vi "run_experiment.vi"(0 "GUI refnum cluster":T34, 1 "all settings":T1={"Variable Settings"={"Measurements per Iteration"=0, "Local Data Path"=path "", "Experiment description suffix for filename (no spaces please)"="", "Network Data Path"=path "", "Copy data to network"=FALSE, "Measurement Timeout (ms)"=0, "Independent Variables"=[], "Dependent Variables"=[], "Run Test Mode"=FALSE}, "HSDIO Settings"={"Enable HSDIO Pulses"=TRUE, "Resource Name"="PXI1Slot6", "Clock Rate"=20000000.0, "Array of Script Triggers"=[], "Channels Control"=[["Hex 3D MOT b0", "1", "0", "", "", "", "", "", "", "", "", "", "", "", "", "", "", "", "", ""], ["Hex 3D MOT b0", "1", "0", "", "", "", "", "", "", "", "", "", "", "", "", "", "", "", "", ""], ["repumper bit0", "1", "0", "", "", "", "", "", "", "", "", "", "", "", "", "", "", "", "", ""], ["Trap Array beam switch", "1", "0", "", "", "", "", "", "", "", "", "", "", "", "", "", "", "", "", ""], ["2D MOT switch", "1", "0", "", "", "", "", "", "", "", "", "", "", "", "", "", "", "", "", ""], ["Hamamatsu CCD trigger", "1", "0", "", "", "", "", "", "", "", "", "", "", "", "", "", "", "", "", ""], ["Luca CCD trigger", "1", "0", "", "", "", "", "", "", "", "", "", "", "", "", "", "", "", "", ""], ["broken", "", "", "", "", "", "", "", "", "", "", "", "", "", "", "", "", "", "", ""], ["repumper bit1", "1", "0", "", "", "", "", "", "", "", "", "", "", "", "", "", "", "", "", ""], ["blow away", "1", "0", "", "", "", "", "", "", "", "", "", "", "", "", "", "", "", "", ""], ["trap shutter", "1", "0", "", "", "", "", "", "", "", "", "", "", "", "", "", "", "", "", ""], ["1038 switch", "1", "0", "", "", "", "", "", "", "", "", "", "", "", "", "", "", "", "", ""], ["", "", "", "", "", "", "", "", "", "", "", "", "", "", "", "", "", "", "", ""], ["", "", "", "", "", "", "", "", "", "", "", "", "", "", "", "", "", "", "", ""], ["", "", "", "", "", "", "", "", "", "", "", "", "", "", "", "", "", "", "", ""], ["", "", "", "", "", "", "", "", "", "", "", "", "", "", "", "", "", "", "", ""], ["", "", "", "", "", "", "", "", "", "", "", "", "", "", "", "", "", "", "", ""], ["", "", "", "", "", "", "", "", "", "", "", "", "", "", "", "", "", "", "", ""], ["", "", "", "", "", "", "", "", "", "", "", "", "", "", "", "", "", "", "", ""], ["", "", "", "", "", "", "", "", "", "", "", "", "", "", "", "", "", "", "", ""], ["", "", "", "", "", "", "", "", "", "", "", "", "", "", "", "", "", "", "", ""], ["", "", "", "", "", "", "", "", "", "", "", "", "", "", "", "", "", "", "", ""], ["", "", "", "", "", "", "", "", "", "", "", "", "", "", "", "", "", "", "", ""], ["", "", "", "", "", "", "", "", "", "", "", "", "", "", "", "", "", "", "", ""], ["", "", "", "", "", "", "", "", "", "", "", "", "", "", "", "", "", "", "", ""], ["", "", "", "", "", "", "", "", "", "", "", "", "", "", "", "", "", "", "", ""], ["", "", "", "", "", "", "", "", "", "", "", "", "", "", "", "", "", "", "", ""], ["", "", "", "", "", "", "", "", "", "", "", "", "", "", "", "", "", "", "", ""], ["", "", "", "", "", "", "", "", "", "", "", "", "", "", "", "", "", "", "", ""], ["", "", "", "", "", "", "", "", "", "", "", "", "", "", "", "", "", "", "", ""], ["", "", "", "", "", "", "", "", "", "", "", "", "", "", "", "", "", "", "", ""]], "Pulse Generation Script"="script script1\n     Generate RedTrap_compress_temp\nend script", "Start Trigger"={"Wait for start trigger?"=FALSE, "source (PFI 0)"="PFI0", "edge (rising)"=12}, "Hardware alignment quantum\n(in samples)"=1, "Inital State"="", "Idle State"="", "Active Channels"="", "Array of Waveforms"=[]}, "DAQmx Pulse Settings"={"Enable DAQmx Pulses"=FALSE, "DAQmx Physical Channels"="", "Clock Rate"=0.0, "units/sec (ms=1000)"=0.0, "Start Trigger"={"Wait for start trigger?"=FALSE, "source"="", "edge"=0}, "Timing Sequence Control"=[]}, "DDS Settings"={"Enable DDS"=FALSE, "Array of DDS Boxes"=[]}, "Camera settings"={"Analog Gain (0-5)"=4, "Exposure Time"=0.01, "EM Gain (0-255)"=0, "Trigger Polarity"="ATP P", "External Trigger Mode"="EMD E", "Scan Speed"="SSP H", "External Trigger Source"="ESC B", "Scan Mode"="SMD N", "Super Pixel Binning\n(if enabled in Scan Mode)"="SPX 1", "Camera Sub-array acquisition region\n(if enabled in scan mode)"={"Left"=0, "Top"=0, "Width"=0, "Height"=0}, "Use camera?"=FALSE, "# image buffers"=100, "shots per measurement"=100, "Force images to U16"=FALSE, "Low Light Sensitivity"="LLS 0", "cooling"="CSW F", "fan"="FAN F", "Frame Grabber acquisition region"={"Left"=0, "Top"=0, "Right"=0, "Bottom"=0}}, "Counter Settings"={"Enable Counters"=FALSE, "Array of Counter Settings"=[]}, "Filter Cluster"={"Counter Filter thresholds"=[], "Data Filters\nROI Minimum Thresholds"=[]}, "Analog Output Parameters"={"Enable Analog Out?"=FALSE, "Physical Channel"="PXI1Slot2/ao0:2", "Minimum Value"=-10.0, "Maximum Value"=10.0, "Samples per second"=0.0, "Total AO Time (seconds)"=0.0, "Start Trigger"={"Wait for start trigger?"=FALSE, "source"="/Dev1/PFI0", "edge"=10280}, "Analog Output Waveforms (channel, time)"=[]}, "Notes"="", "HP83623A Generator Settings Array"=[], "Iteration Graph Settings"={"Plot Regions"="", "Plot Shots"=""}, "PI Piezo Settings"={"Enable"=FALSE, "Array of Piezo Controllers"=[]}, "Andor settings"={"Andor Path"=path "", "Copy any Andor files"=FALSE, "Wait time before copying Andor files (ms)"=0}, "Measurement Chart Settings"={"Which regions to plot (comma separated)"="", "Which shot to plot"=0}, "HP8662A Synthesized Signal Generator Array"=[], "HP83712B Synthesized CW Generator Array"=[], "TTL input"={"Enable"=FALSE, "lines"=""}} {"Variable Settings"."Independent Variables"."# steps" min=1 step=1; "Variable Settings"."Measurements per Iteration" min=1 step=1; "HSDIO Settings"."Hardware alignment quantum\n(in samples)" min=1 step=1; "HSDIO Settings"."Array of Script Triggers"."level" items=["High Level"=34, "Low Level"=35]; "HSDIO Settings"."Array of Script Triggers"."edge" items=["Rising Edge"=12, "Falling Edge"=13]; "HSDIO Settings"."Start Trigger"."edge (rising)" items=["Rising Edge"=12, "Falling Edge"=13]; "HSDIO Settings"."Clock Rate" min=0.0 max=200000000.0 format="%.2p"; "DAQmx Pulse Settings"."Start Trigger"."edge" items=["Rising"=10280, "Falling"=10171]; "DAQmx Pulse Settings"."Clock Rate" min=0.0 max=200000000.0 format="%.2p"; "Camera settings"."Frame Grabber acquisition region"."Bottom" max=512 step=1; "Camera settings"."Frame Grabber acquisition region"."Right" max=512 step=1; "Camera settings"."Frame Grabber acquisition region"."Top" max=512 step=1; "Camera settings"."Frame Grabber acquisition region"."Left" max=512 step=1; "Camera settings"."shots per measurement" min=0 step=1; "Camera settings"."# image buffers" min=0 step=1; "Camera settings"."Camera Sub-array acquisition region\n(if enabled in scan mode)"."Height" min=16 max=512 step=16; "Camera settings"."Camera Sub-array acquisition region\n(if enabled in scan mode)"."Width" min=16 max=512 step=16; "Camera settings"."Camera Sub-array acquisition region\n(if enabled in scan mode)"."Top" max=496 step=16; "Camera settings"."Camera Sub-array acquisition region\n(if enabled in scan mode)"."Left" max=496 step=16; "Camera settings"."Analog Gain (0-5)" max=5 step=1; "Counter Settings"."Array of Counter Settings"."Binwidth (ms)" format="%0.2f"; "Analog Output Parameters"."Start Trigger"."edge" items=["Rising"=10280, "Falling"=10171]; "Analog Output Parameters"."Maximum Value" format="%0.2f"; "Analog Output Parameters"."Minimum Value" format="%0.2f"}, 2 "Variable Settings Refnum":refnum<vi>, 7 "error in (no error)":errorcluster, 8 "Image Display Refnum Array":refnum<vi>[](array[refnum]), 12 "Camera Temperature Refnum":refnum<vi>, 14 "HSDIO Status Refnum":refnum<vi>, 16 "# intervals (mutli-shot)":i32=128, 17 "Notes Refnum":refnum<vi>, 22 "Hamamatsu_C9100-13.lvclass":refnum<class "Hamamatsu_C9100-13.lvclass">) -> (20 "Array of ROI sums":dbl[][][][](array[numeric])=[[[[-878.86977886979]]]], 21 "Image Array for whole experiment":T39[][][](array[plugin-control]) caption="(Cycles, Iterations, Measurements, Shots, scaling above)", 23 "Histogram of ROI Sum over All Images for last ROI":T37, 24 "Average of All Images from experiment":T39(plugin-control) caption="Average of All Images (dynamically scaled)", 25 "Camera out":refnum<class "Hamamatsu_C9100-13.lvclass">, 27 "error out":errorcluster)   [LabVIEW 2013]
doc: "I Description:\nThis example uses a script to manage the generation of a dynamic pattern at a specified clock rate.\n\nII Instructions for Running:\n1. Enter the digital channels on the hardware device to generate digital pattern in the Channel List control.\n2. Specify the clock rate for the generation in the Clock Rate control.\n3. Click the Stop button when you want to stop the generation\n\nIII Block Diagram Steps:\n1. Initialize for a generation session.\n2. Assign specified channels in Channel List for dynamic operation.\n3. Configure the Sample clock to use the onboard clock, and configure the clock rate.\n4. Set the generation mode to Scripted.\n5. Query the Data Width property to determine which Write function to use.\nNote: Different devices have different default values for the Data Width property. If you know the Data Width of your device, you may omit the property node and case structure.\n6. Write digital patterns to the onboard memory of the digital device.\n7. Write the script to the onboard memory.\n8. Initiate dynamic pattern generation.\n9. Wait until the Stop button is clicked or an error occurs, and exit the While loop. \n The niHSDIO Is Done VI is used in the while loop to check only for errors.\n10. Abort generation and close the session.\n\nIV I/O Connections Overview:\nMake connections from output terminals to match the channels specified by Channel List. In this example, the digital pattern is generated from the first 16 digital channels of the device."
uses:
  Camera/Hamamatsu_C9100-13/Hamamatsu_C9100-13.lvclass
  ExperimentVariables/ExperimentVariables.lvclass
  DDS/DDS.lvclass
  PI_piezo/PI_Piezo.lvclass
  HSDIO/HSDIO.lvclass
  DAQmx_pulse_out/DAQmx_pulse_out.lvclass
  Analog_output/Analog_Output.lvclass
  Counter/Counter.lvclass
  GPIB/GPIB.lvclass
  TTL_input/TTL_input.lvclass
  Analog_output/AO_settings.ctl
  Camera/Hamamatsu_C9100-13/camera_setup.ctl
  DDS drivers v3/DDS RAM mode.ctl
  <vilib>/ni845x/ni845x.llb/ni845xControl.ctl
  <instrlib>/niHSDIO/niHSDIO.llb/niHSDIO_ctl Trigger Script - trigID Values (Ring).ctl
  <instrlib>/niHSDIO/niHSDIO.llb/niHSDIO_ctl Trigger DigEdge - Edge Values (Ring).ctl
  <instrlib>/niHSDIO/niHSDIO.llb/niHSDIO_ctl Trigger Source Values (Ring).ctl
  ExperimentVariables/Variable_Settings.ctl
  Counter/Counter_Settings_Control.ctl
  HSDIO/HSDIO_settings.ctl
  DAQmx_pulse_out/settings.ctl
  <instrlib>/niHSDIO/niHSDIO.llb/niHSDIO_ctl Trigger DigLvl - Level Values (Ring).ctl
  histogram.ctl
  gui_refnum.ctl
  Counter/counter_graph_refnums.ctl
  filters/filters.ctl
  gui_execution_controls.ctl
  DDS drivers v3/Array_of_DDS_Boxes.ctl
  DDS drivers v3/DDS_box_device_reference.ctl
  DDS drivers v3/DDS_box_cluster.ctl
  DDS/DDS_Settings_Cluster.ctl
  config_file_io/all_settings.ctl
  GPIB/HP83623A_RF_Generator/HP83623A_array.ctl
  GPIB/HP83623A_RF_Generator/HP83623A_RF_Generator.lvclass
  PI_piezo/settings.ctl
  PI_piezo/status.ctl
  Camera/Andor/Andor_settings.ctl
  gui/measurement_graph.ctl
  GPIB/RF_Generator_settings.ctl
  GPIB/RF_Generator_settings_array.ctl
  DDS drivers v3/DDS_profile.ctl
  DDS drivers v3/DDS_channel.ctl
  DDS drivers v3/array_of_DDS_profiles.ctl
  DDS drivers v3/array_of_DDS_channels.ctl
  TTL_input/TTL_input_settings.ctl
  HSDIO/waveform.ctl
  PI_piezo/piezo_channel.ctl
  PI_piezo/piezo_controller.ctl
  GPIB/HP83623A_RF_Generator/HP83623A.ctl
panel:
  out "Counter out":refnum<class "Counter.lvclass">
  out "HSDIO":refnum<class "HSDIO.lvclass">
  out "Run Test Mode":bool
  in  "Tab Control":T38(tab)=enum."Filters"
  # "Parameters will be evaluated once at the beginning of the experiment from top to bottom, \nso any parameter may depend on all those above it.\nVariables will be evaluated each iteration.\nParameters and Variables may be used in various other experiment settings, as noted.\nSee LabView Help -> Formula Node and Expression Node Functions for a list of available functions."
  # "Parameters will be evaluated once at the beginning of the experiment from top to bottom, \nso any parameter may depend on all those above it.\nVariables will be evaluated each iteration.\nParameters and Variables may be used in various other experiment settings, as noted.\nSee LabView Help -> Formula Node and Expression Node Functions for a list of available functions."
  # "Regions of Interest -->"
  # "Shots\n   |\n  V"
  # "Counters -->"
  # "Counter\n    bins\n       |\n      V"
  # "Notes will be auto-evaluated and will be saved with comments in each experiment directory."
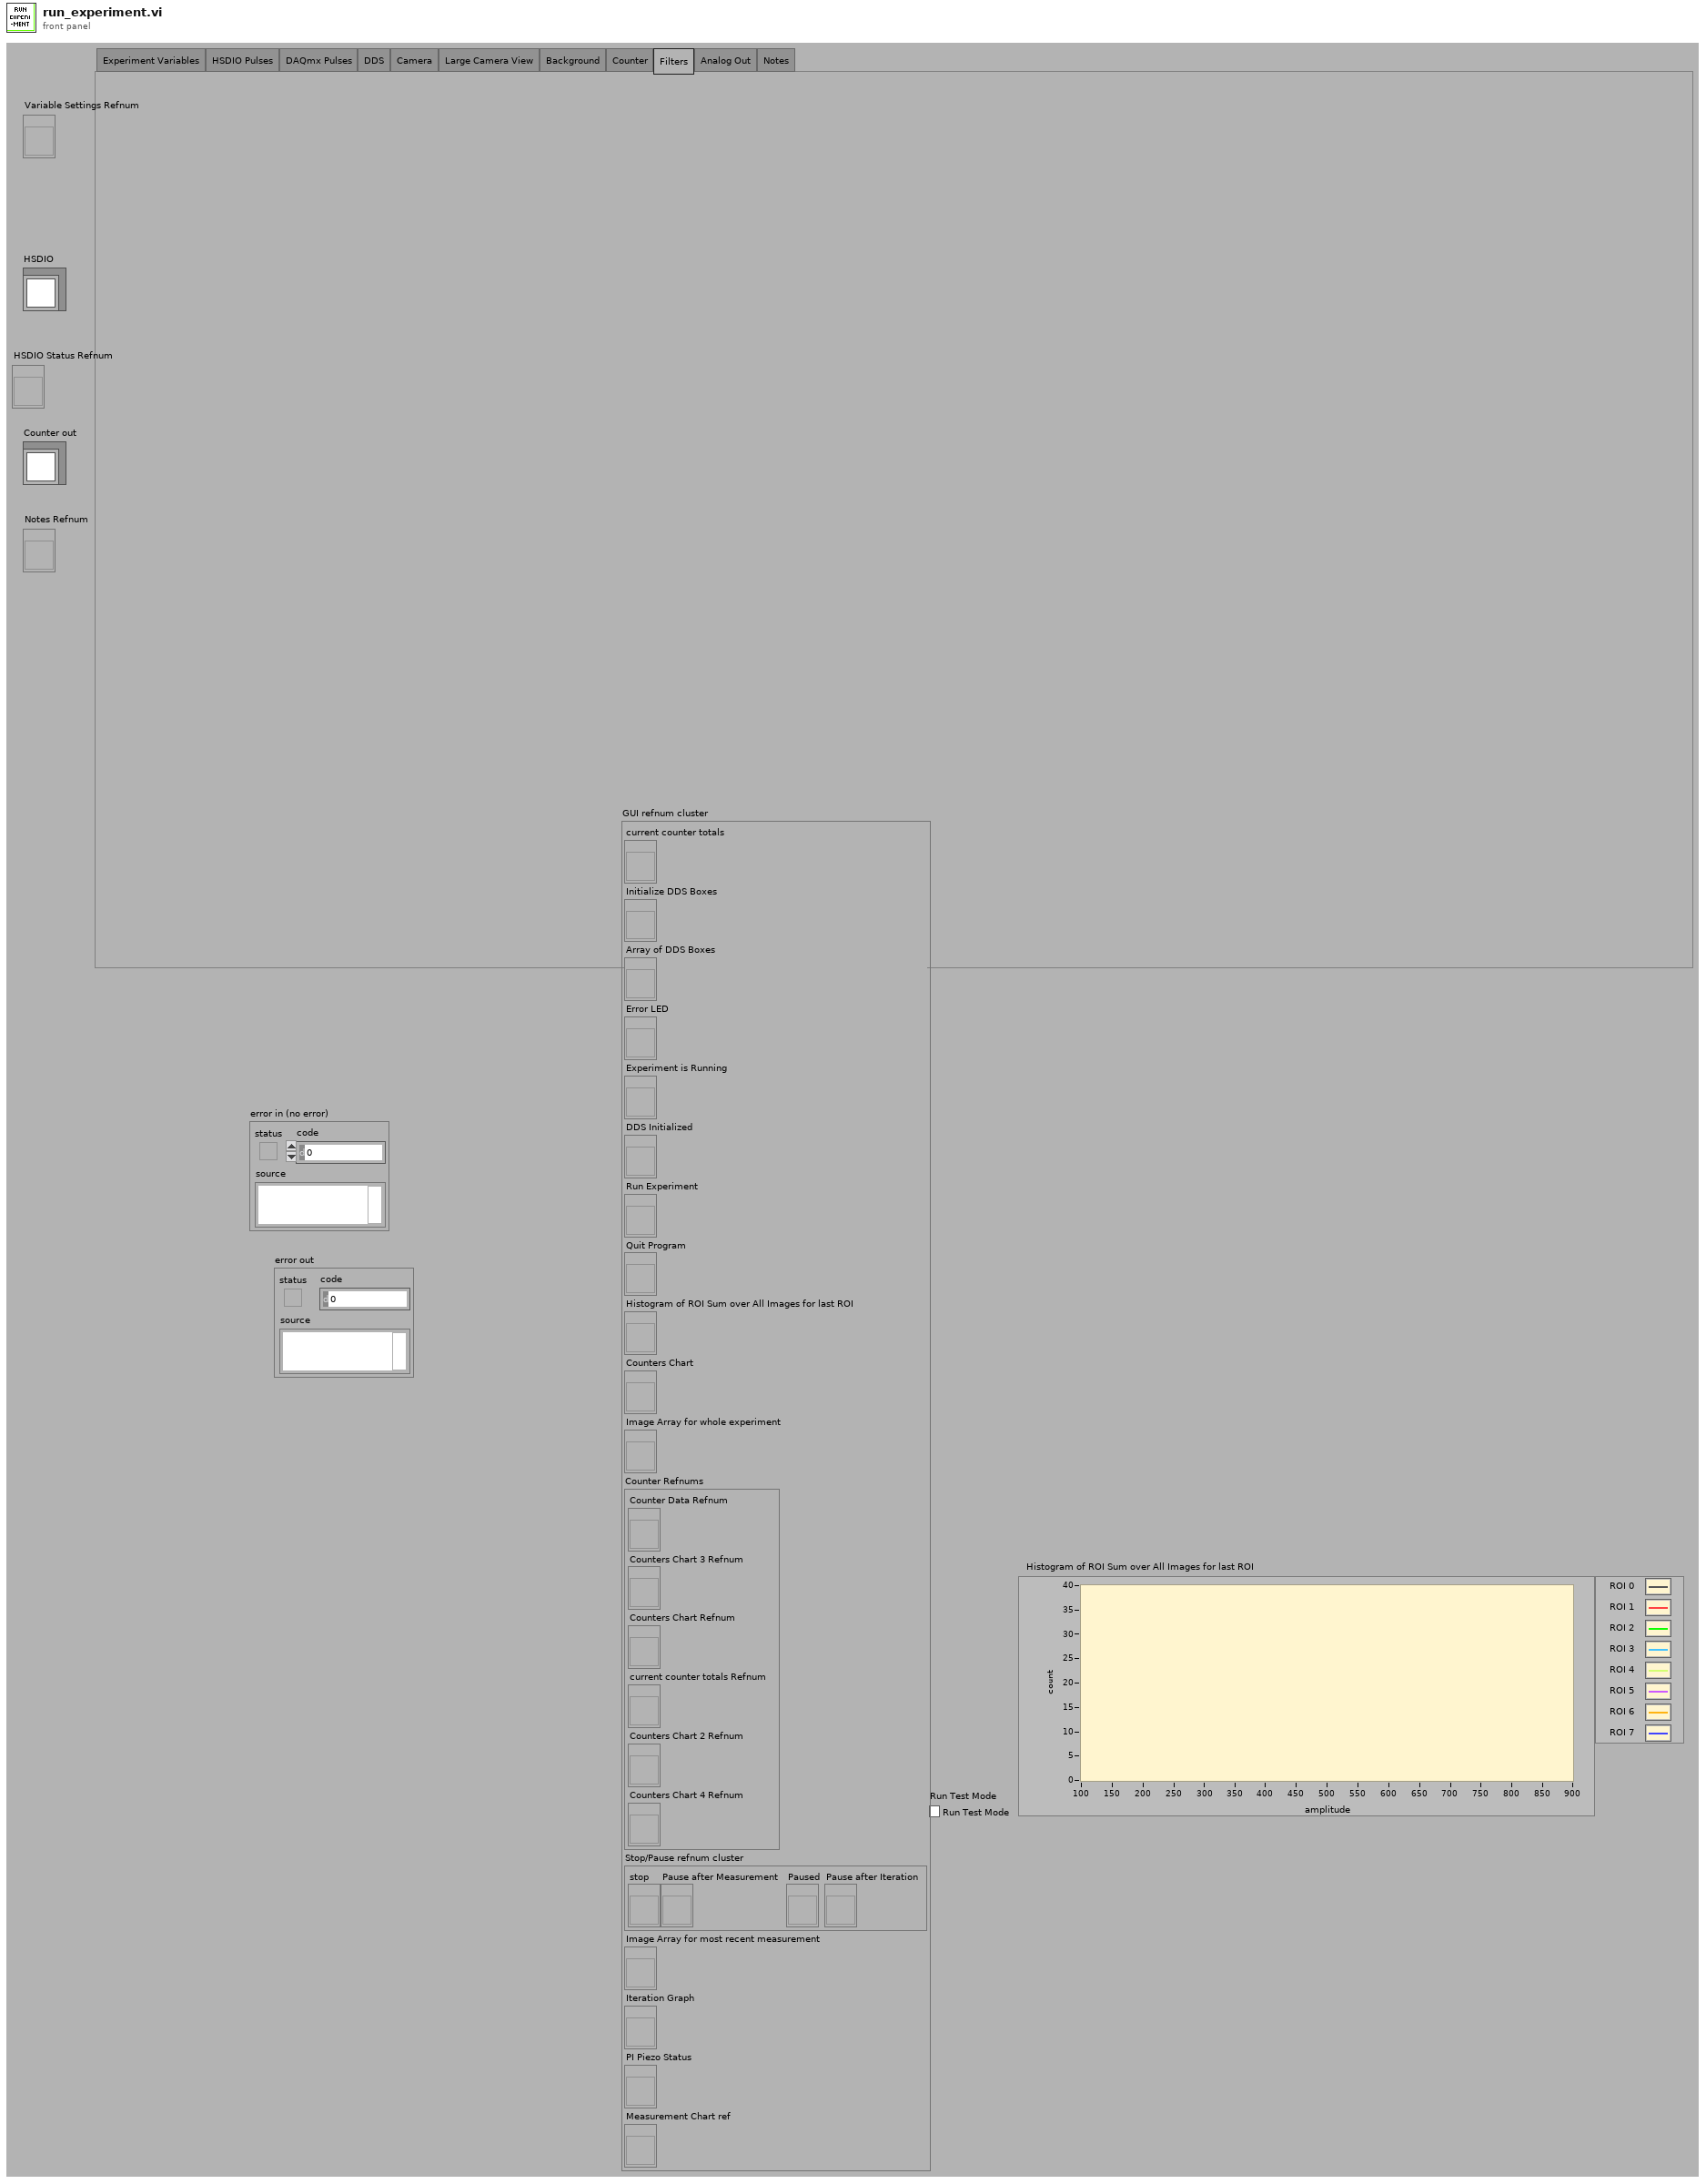
[diagram p1: front panel]
types:
  T1 = typedef "all_settings.ctl" = cluster{"Variable Settings":T2, "HSDIO Settings":T3, "DAQmx Pulse Settings":T9, "DDS Settings":T10, "Camera settings":T20, "Counter Settings":T21, "Filter Cluster":T22, "Analog Output Parameters":T23, "Notes":string, "HP83623A Generator Settings Array":T24, "Iteration Graph Settings":cluster{"Plot Regions":string, "Plot Shots":string}, "PI Piezo Settings":T26, "Andor settings":T29, "Measurement Chart Settings":T30, "HP8662A Synthesized Signal Generator Array":T31, "HP83712B Synthesized CW Generator Array":T31, "TTL input":T33}
  T2 = typedef "ExperimentVariables.lvclass/Variable_Settings.ctl" = cluster{"Measurements per Iteration":i32, "Local Data Path":path, "Experiment description suffix for filename (no spaces please)":string, "Network Data Path":path, "Copy data to network":bool, "Measurement Timeout (ms)":u32, "Independent Variables":cluster{"Description":string, "Name (a,a0...a9)":string, "min":dbl, "max":dbl, "# steps":u32}[], "Dependent Variables":cluster{"Description":string, "Name (a,a0...a9)":string, "Equation":string, "Result":dbl}[], "Run Test Mode":bool}
  T3 = typedef "HSDIO.lvclass/HSDIO_settings.ctl" = cluster{"Enable HSDIO Pulses":bool, "Resource Name":refnum<k15>, "Clock Rate":dbl, "Array of Script Triggers":cluster{"trigger id (script trigger 0)":T4, "source (PFI 0)":T5, "Trigger Type":enum32{"Edge", "Level"}, "edge":T6, "level":T7}[], "Channels Control":string[][], "Pulse Generation Script":string, "Start Trigger":cluster{"Wait for start trigger?":bool, "source (PFI 0)":T5, "edge (rising)":T6}, "Hardware alignment quantum\n(in samples)":u16, "Inital State":string, "Idle State":string, "Active Channels":string, "Array of Waveforms":T8[]}
  T4 = typedef "niHSDIO_ctl Trigger Script - trigID Values (Ring).ctl" = string
  T5 = typedef "niHSDIO_ctl Trigger Source Values (Ring).ctl" = string
  T6 = typedef "niHSDIO_ctl Trigger DigEdge - Edge Values (Ring).ctl" = i32
  T7 = typedef "niHSDIO_ctl Trigger DigLvl - Level Values (Ring).ctl" = i32
  T8 = typedef "HSDIO.lvclass/waveform.ctl" = cluster{"name":string, "transitions":u32[], "states":u8[][]}
  T9 = typedef "DAQmx_pulse_out.lvclass/settings.ctl" = cluster{"Enable DAQmx Pulses":bool, "DAQmx Physical Channels":tag, "Clock Rate":dbl, "units/sec (ms=1000)":dbl, "Start Trigger":cluster{"Wait for start trigger?":bool, "source":tag, "edge":i32}, "Timing Sequence Control":string[][]}
  T10 = typedef "DDS_Settings_Cluster.ctl" = cluster{"Enable DDS":bool, "Array of DDS Boxes":T11}
  T11 = typedef "Array_of_DDS_Boxes.ctl" = T12[]
  T12 = typedef "DDS_box_cluster.ctl" = cluster{"DDS box device reference":T13, "Array of DDS Channels (4)":T15, "Enable":bool, "Description":string}
  T13 = typedef "DDS_box_device_reference.ctl" = cluster{"NI USB-8451 device reference":T14, "DIO port":u8, "Serial Clock Rate [kHz]":u16}
  T14 = typedef "ni845xControl.ctl" = refnum<k21>
  T15 = typedef "DDS.lvclass/array_of_DDS_channels.ctl" = T16[]
  T16 = typedef "DDS.lvclass/DDS_channel.ctl" = cluster{"Power":bool, "Channel Parameters":cluster{"Ref Clock Rate [kHz]":dbl, "Full Scale Output\nPower [dBm]":dbl}, "RAM Enable":bool, "RAM Dest Type":u8, "RAM Default":cluster{"Frequency [MHz]":dbl, "Amplitude [dBm]":dbl, "Phase Offset [rad]":dbl}, "Array of DDS Profiles (8)":T17, "Description":string}
  T17 = typedef "DDS.lvclass/array_of_DDS_profiles.ctl" = T18[]
  T18 = typedef "DDS_profile.ctl" = cluster{"Single Tone":cluster{"Frequency [MHz]":dbl, "Amplitude [dBm]":dbl, "Phase Offset [rad]":dbl}, "RAM Mode ":T19, "Zero-crossing":bool, "No Dwell High":bool, "Function/Static":bool, "RAM Function Settings":string[], "RAM Static Array":dbl[], "Description":string}
  T19 = typedef "DDS RAM mode.ctl" = enum16{"Direct Switch", "Ramp Up", "Bidirectional Ramp", "Continuous Bidirectional Ramp", "Continuous Recirculate", "Direct Switch 2", "Direct Switch 3", "Direct Switch 4"}
  T20 = typedef "Hamamatsu_C9100-13.lvclass/camera_setup.ctl" = cluster{"Analog Gain (0-5)":u8, "Exposure Time":dbl, "EM Gain (0-255)":u8, "Trigger Polarity":string, "External Trigger Mode":string, "Scan Speed":string, "External Trigger Source":string, "Scan Mode":string, "Super Pixel Binning\n(if enabled in Scan Mode)":string, "Camera Sub-array acquisition region\n(if enabled in scan mode)":cluster{"Left":u16, "Top":u16, "Width":u16, "Height":u16}, "Use camera?":bool, "# image buffers":i32, "shots per measurement":i32, "Force images to U16":bool, "Low Light Sensitivity":string, "cooling":string, "fan":string, "Frame Grabber acquisition region":cluster{"Left":i32, "Top":i32, "Right":i32, "Bottom":i32}}
  T21 = typedef "Counter.lvclass/Counter_Settings_Control.ctl" = cluster{"Enable Counters":bool, "Array of Counter Settings":cluster{"Counter Channel":tag, "Time-Bin Clock Channel":tag, "Binwidth (ms)":dbl}[]}
  T22 = typedef "filters.ctl" = cluster{"Counter Filter thresholds":u32[][], "Data Filters\nROI Minimum Thresholds":u64[][]}
  T23 = typedef "Analog_Output.lvclass/AO_settings.ctl" = cluster{"Enable Analog Out?":bool, "Physical Channel":tag, "Minimum Value":dbl, "Maximum Value":dbl, "Samples per second":dbl, "Total AO Time (seconds)":dbl, "Start Trigger":cluster{"Wait for start trigger?":bool, "source":tag, "edge":i32}, "Analog Output Waveforms (channel, time)":dbl[][]}
  T24 = typedef "HP83623A_RF_Generator.lvclass/HP83623A_array.ctl" = T25[]
  T25 = typedef "HP83623A_RF_Generator.lvclass/HP83623A.ctl" = cluster{"Frequency (Hz)":dbl, "Power (dBm)":dbl, "Enabled":bool, "initialized":bool, "RF Output On/Off":bool, "External Trigger?":bool, "VISA Session":refnum<visa-resource-name>, "Generator Name":string}
  T26 = typedef "PI_Piezo.lvclass/settings.ctl" = cluster{"Enable":bool, "Array of Piezo Controllers":T27[]}
  T27 = typedef "PI_Piezo.lvclass/piezo_controller.ctl" = cluster{"Enable":bool, "Serial No.":string, "Array of Piezo Channels":T28[]}
  T28 = typedef "PI_Piezo.lvclass/piezo_channel.ctl" = cluster{"Servo":bool, "Set Position":dbl}
  T29 = typedef "Andor_settings.ctl" = cluster{"Andor Path":path, "Copy any Andor files":bool, "Wait time before copying Andor files (ms)":u16}
  T30 = typedef "measurement_graph.ctl" = cluster{"Which regions to plot (comma separated)":string, "Which shot to plot":u8}
  T31 = typedef "GPIB.lvclass/RF_Generator_settings_array.ctl" = T32[]
  T32 = typedef "GPIB.lvclass/RF_Generator_settings.ctl" = cluster{"Enable":bool, "Description":string, "GPIB channel #":u8, "Frequency (MHz)":dbl, "Power (dBm)":dbl}
  T33 = typedef "TTL_input.lvclass/TTL_input_settings.ctl" = cluster{"Enable":bool, "lines":tag}
  T34 = typedef "gui_refnum.ctl" = cluster{"current counter totals":refnum<vi>, "Initialize DDS Boxes":refnum<vi>, "Array of DDS Boxes":refnum<vi>, "Error LED":refnum<vi>, "Experiment is Running":refnum<vi>, "DDS Initialized":refnum<vi>, "Run Experiment":refnum<vi>, "Quit Program":refnum<vi>, "Histogram of ROI Sum over All Images for last ROI":refnum<vi>, "Counters Chart":refnum<vi>, "Image Array for whole experiment":refnum<vi>, "Counter Refnums":T35, "Stop/Pause refnum cluster":T36, "Image Array for most recent measurement":refnum<vi>, "Iteration Graph":refnum<vi>, "PI Piezo Status":refnum<vi>, "Measurement Chart ref":refnum<vi>}
  T35 = typedef "counter_graph_refnums.ctl" = cluster{"Counter Data Refnum":refnum<vi>, "Counters Chart 3 Refnum":refnum<vi>, "Counters Chart Refnum":refnum<vi>, "current counter totals Refnum":refnum<vi>, "Counters Chart 2 Refnum":refnum<vi>, "Counters Chart 4 Refnum":refnum<vi>}
  T36 = typedef "gui_execution_controls.ctl" = cluster{"stop":refnum<vi>, "Pause after Measurement":refnum<vi>, "Paused":refnum<vi>, "Pause after Iteration":refnum<vi>}
  T37 = typedef "histogram.ctl" = cluster{"X Values":dbl[], "Histogram: h(x)":i32[]}[]
  T38 = enum32{"Experiment Variables", "HSDIO Pulses", "DAQmx Pulses", "DDS", "Camera", "Large Camera View", "Background", "Counter", "Filters", "Analog Out", "Notes"}
  T39 = typedef "IMAQ Image.ctl" = refnum<image>
  T40 = enum16{"reset", "experiment start", "experiment end", "quit"}
  T41 = cluster{"Plot Regions":string, "Plot Shots":string}
  T42 = cluster{"X Values":dbl[], "Histogram: h(x)":i32[]}[]
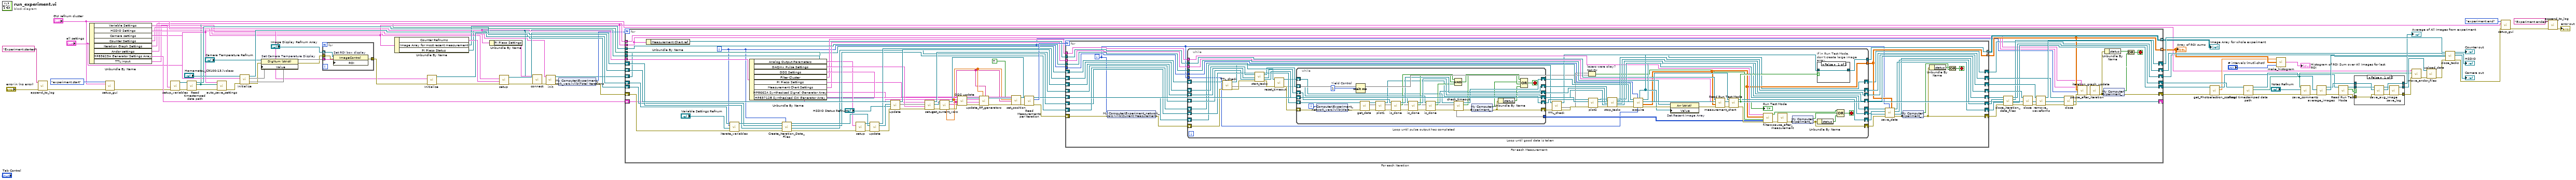
[diagram p0: block diagram]
diagram:
  n1 = call "append_to_log.vi"("error in"="error in (no error)", "string"="Experiment started") -> ("error out"=w58:errorcluster)  [unwired: 9 in]
  n2 = Unbundle By Name("all settings") -> ("Variable Settings"=w25:T2, "HSDIO Settings"=w24:T3, "Camera settings"=w23:T20, "Counter Settings"=w22:T21, "Iteration Graph Settings"=w19:T41, "Andor settings"=w11:T29, "HP83623A Generator Settings Array"=w9:T24, "TTL input"=w5:T33)
  n3 = call "setup_gui.vi"("Enum"=T40."experiment start", "GUI refnum cluster"="GUI refnum cluster", "error in (no error)"=w58) -> ("error out"=w8:errorcluster)  [unwired: 12 in]
  n4 = call "setup_variables.vi"("error in (no error)"=w8, "Variable Settings"=w25) -> ("error out"=w45:errorcluster, "ExperimentVariables out"=w47:refnum<class "ExperimentVariables.lvclass">)  [unwired: 8 in]
  n5 = call-dynamic "Read timestamped data path.vi"("error in (no error)"=w45, "ExperimentVariables in"=w47) -> ("error out"=w26:errorcluster, "Specific Data Files Path"=w14:path, "ExperimentVariables out"=w46:refnum<class "ExperimentVariables.lvclass">)  [unwired: 7 in]
  n6 = call "auto_save_settings.vi"("error in"=w26, "base path"=w14, "all settings"="all settings") -> ("error out"=w21:errorcluster)  [unwired: 8 in]
  n7 = call-dynamic "initialize.vi"("error in (no error)"=w21, 10:w23, "Hamamatsu_C9100-13 in"="Hamamatsu_C9100-13.lvclass") -> ("error out"=w62:errorcluster, 2:w63, "Hamamatsu_C9100-13 out"=w69:refnum<class "Hamamatsu_C9100-13.lvclass">, 6:w70)  [unwired: 5 in]
  n8 = property on="Set Camera Temperature Display" class="DigNum (strict)"(reference="Camera Temperature Refnum", error in=w62, "Value"=w63) -> (error out=w61:errorcluster)  [unwired: 1 out]
  n9 = for {
    tunnel: "Image Display Refnum Array" -> [w84] mode=indexing
    tunnel: w70 -> [w83]
    tunnel: w61 -> [w82]
    tunnel: [w81] -> w71
    n10 = property on="Set ROI box display" class="ImageControl"(reference=w84, error in=w82, "ROI"=w83) -> (error out=w81:errorcluster)  [unwired: 1 out]
  }
  n11 = Unbundle By Name("GUI refnum cluster") -> ("Counter Refnums"=w28:T35, "Image Array for most recent measurement"=w27:refnum<vi>, "PI Piezo Status"=w15:refnum<vi>)
  n12 = call "Initialize.vi"("error in (no error)"=w71, 10:w24) -> ("error out"=w54:errorcluster, "HSDIO out"=w75:refnum<class "HSDIO.lvclass">)  [unwired: 8 in]
  n13 = Unbundle By Name("all settings") -> ("PI Piezo Settings"=w16:T26)
  n14 = call "setup.vi"("error in (no error)"=w54, "Counter Refnums"=w28, "Counter Settings"=w22) -> ("error out"=w18:errorcluster, "Counter out"=w53:refnum<class "Counter.lvclass">)  [unwired: 7 in]
  n15 = call "connect.vi"(0:w16, 1:w15, "error in"=w18) -> ("error out"=w4:errorcluster)  [unwired: 16 in]
  n16 = call "init.vi"("error in (no error)"=w4, "TTL input"=w5) -> ("error out"=w3:errorcluster, "TTL_input out"=w2:refnum<class "TTL_input.lvclass">)  [unwired: 8 in]
  n17 = shared-variable "My Computer\\Experiment_network_vars.lvlib\\Total Iterations"(error in=w3) -> (w7:u32, error out=w6:errorcluster)
  n18 = for "For each Iteration" {
    N: w7 -> [_]
    shift-right: [w89] -> w33
    shift-left: w6 -> [w159]
    tunnel: [w111] -> w67 mode=indexing
    shift-right: [w155] -> w76
    shift-left: w75 -> [w158]
    shift-right: [w121] -> w77
    shift-left: w53 -> [w131]
    shift-right: [w124] -> w50
    shift-left: w46 -> [w160]
    tunnel: [w136] -> w74 mode=indexing
    shift-right: [w112] -> w34
    shift-left: w69 -> [w130]
    tunnel: w27 -> [w120]
    tunnel: "all settings" -> [w119]
    tunnel: "GUI refnum cluster" -> [w101]
    tunnel: w19 -> [w108]
    tunnel: w15 -> [w106]
    tunnel: w14 -> [w102]
    shift-right: [w92] -> _
    shift-left: w9 -> [w93]
    shift-right: [w87] -> w1
    shift-left: w2 -> [w88]
    i -> [w85]
    stop <- w162 stop-if-true
    n19 = Unbundle By Name(w101) -> ("Measurement Chart ref"=w100:refnum<vi>)
    n20 = call-dynamic "iterate_variables.vi"("error in (no error)"=w159, "Variable Settings Refnum"="Variable Settings Refnum", "Current Iteration"=w85, "ExperimentVariables in"=w160) -> ("error out"=w133:errorcluster, "ExperimentVariables out"=w135:refnum<class "ExperimentVariables.lvclass">)  [unwired: 6 in]
    n21 = Unbundle By Name(w119) -> ("Analog Output Parameters"=w116:T23, "DAQmx Pulse Settings"=w117:T9, "DDS Settings"=w118:T10, "Filter Cluster"=w115:T22, "PI Piezo Settings"=w107:T26, "Measurement Chart Settings"=w99:T30, "HP8662A Synthesized Signal Generator Array"=w98:T31, "HP83712B Synthesized CW Generator Array"=w86:T31)
    n22 = call-dynamic "Create_Iteration_Data_Files.vi"("Current Iteration"=w85, "error in (no error)"=w133, "Counter (in)"=w131, "Hamamatsu_C9100-13 (in)"=w130, "ExperimentVariables in"=w135) -> ("error out"=w132:errorcluster, "Counter out"=w128:refnum<class "Counter.lvclass">, "Hamamatsu_C9100-13"=w129:refnum<class "Hamamatsu_C9100-13.lvclass">, "ExperimentVariables out"=w134:refnum<class "ExperimentVariables.lvclass">)  [unwired: 3 in]
    n23 = call "setup.vi"("error in (no error)"=w132, "Analog Output Parameters"=w116) -> ("error out"=w137:errorcluster, "Analog_Output out"=w138:refnum<class "Analog_Output.lvclass">)  [unwired: 8 in]
    n24 = call-dynamic "update.vi"("error in (no error)"=w137, "ExperimentVariables (in)"=w134, "Analog_Output in"=w138) -> ("error out"=w143:errorcluster, "ExperimentVariables"=w141:refnum<class "ExperimentVariables.lvclass">, "Analog_Output out"=w142:refnum<class "Analog_Output.lvclass">)  [unwired: 6 in]
    n25 = call-dynamic "update.vi"("error in (no error)"=w143, 9:"HSDIO Status Refnum", 10:w141, "HSDIO in"=w158) -> ("error out"=w113:errorcluster, 2:w152, "HSDIO out"=w157:refnum<class "HSDIO.lvclass">)  [unwired: 5 in]
    n26 = call "setup.vi"("error in (no error)"=w113, "DAQmx Pulse Settings"=w117, "ExperimentVariables (in)"=w152) -> ("error out"=w153:errorcluster, "ExperimentVariables"=w151:refnum<class "ExperimentVariables.lvclass">, "DAQmx_pulse_out out"=w150:refnum<class "DAQmx_pulse_out.lvclass">)  [unwired: 6 in]
    n27 = call-dynamic "get_current_vars.vi"("error in (no error)"=w153, "ExperimentVariables in"=w151) -> ("error out"=w154:errorcluster, "variables and parameter names"=w94:string[], "ExperimentVariables out"=w145:refnum<class "ExperimentVariables.lvclass">, "current variable and parameter values"=w95:dbl[])  [unwired: 4 in, 2 out]
    n28 = call "DDS update.vi"("error in (no error)"=w154, 9:w94, 10:w95, "DDS.lvclass (in)"=w118) -> ("error out"=w97:errorcluster)  [unwired: 6 in, 1 out]
    n29 = call "update_RF_generators.vi"(5:w94, 7:w95, "error in"=w97, 9:w86, 10:w98, "GPIB (in)"=w93) -> ("error out"=w96:errorcluster, "GPIB"=w92:refnum<class "GPIB.lvclass">)  [unwired: 4 in]
    n30 = call "set_position.vi"(0:w107, 1:w106, 2:w95, 3:w94, "error in"=w96, 6:w102, 8:TRUE ("Save positions?")) -> ("error out"=w105:errorcluster)  [unwired: 12 in]
    n31 = call-dynamic "Read Measurements per Iteration.vi"("error in (no error)"=w105, "ExperimentVariables in"=w145) -> ("error out"=w146:errorcluster, "Measurements per Iteration"=w147:i32, "ExperimentVariables out"=w144:refnum<class "ExperimentVariables.lvclass">)  [unwired: 7 in]
    n32 = for "For each Measurement" {
      N: w147 -> [_]
      shift-right: [w194] -> w156
      shift-left: w157 -> [w195]
      shift-right: [w170] -> w127
      shift-left: w146 -> [w168]
      tunnel: [w184] -> w136 mode=indexing
      tunnel: [w185] -> w111 mode=indexing
      shift-right: [w186] -> w140
      shift-left: w142 -> [w187]
      shift-right: [w180] -> w122
      shift-left: w128 -> [w190]
      shift-right: [w188] -> w149
      shift-left: w150 -> [w189]
      shift-right: [w177] -> w125
      shift-left: w144 -> [w169]
      shift-right: [w178] -> w123
      shift-left: w129 -> [w193]
      tunnel: w120 -> [w176]
      tunnel: w115 -> [w175]
      tunnel: w100 -> [w174]
      tunnel: w99 -> [w173]
      shift-right: [w165] -> w87
      shift-left: w88 -> [w166]
      tunnel: w85 -> [w164]
      i -> [w163]
      stop <- w191 stop-if-true
      n33 = shared-variable "My Computer\\Experiment_network_vars.lvlib\\Current Measurement"(w163, error in=w168) -> (error out=w167:errorcluster)
      n34 = while "Loop until good data is taken" {
        tunnel: [w224] -> w184
        tunnel: [w213] -> w185
        shift-right: [w251] -> w194
        shift-left: w195 -> [w253]
        shift-right: [w210] -> w182
        shift-left: w167 -> [w204]
        shift-right: [w237] -> w186
        shift-left: w187 -> [w236]
        shift-right: [w247] -> w181
        shift-left: w190 -> [w249]
        shift-right: [w243] -> w188
        shift-left: w189 -> [w246]
        shift-right: [w221] -> w183
        shift-left: w169 -> [w240]
        shift-right: [w223] -> w179
        shift-left: w193 -> [w234]
        tunnel: w176 -> [w219]
        tunnel: w175 -> [w218]
        tunnel: w174 -> [w217]
        tunnel: w173 -> [w214]
        shift-right: [w209] -> w165
        shift-left: w166 -> [w205]
        tunnel: w164 -> [w197]
        tunnel: w163 -> [w196]
        stop <- w254 stop-if-true
        n35 = call-dynamic "TTL_check.vi"("error in (no error)"=w204, "TTL_input in"=w205) -> ("error out"=w203:errorcluster, 1:w200, "TTL_input out"=w202:refnum<class "TTL_input.lvclass">)  [unwired: 7 in]
        n36 = call "start_tasks.vi"("Counter (in)"=w249, "Analog_Output in"=w236, "HSDIO (in)"=w253, "DAQmx_pulse_out (in)"=w246, "error in"=w203) -> ("Counter out"=w248:refnum<class "Counter.lvclass">, "Analog_Output"=w235:refnum<class "Analog_Output.lvclass">, "HSDIO"=w250:refnum<class "HSDIO.lvclass">, "DAQmx_pulse_out"=w245:refnum<class "DAQmx_pulse_out.lvclass">, "error out"=w242:errorcluster)  [unwired: 10 in]
        n37 = call-dynamic "reset_timeout.vi"("error in (no error)"=w242, "ExperimentVariables in"=w240) -> ("error out"=w241:errorcluster, "ExperimentVariables out"=w239:refnum<class "ExperimentVariables.lvclass">)  [unwired: 8 in]
        n38 = while "Loop until pulse output has completed" {
          shift-right: [w262] -> w208
          shift-left: w241 -> [w259]
          shift-right: [w284] -> w252
          shift-left: w250 -> [w285]
          shift-right: [w267] -> w229
          shift-left: w248 -> [w269]
          shift-right: [w282] -> w244
          shift-left: w245 -> [w283]
          shift-right: [w274] -> w238
          shift-left: w235 -> [w275]
          shift-right: [w280] -> w232
          shift-left: w239 -> [w260]
          tunnel: [w257] -> w206
          i -> [w261]
          stop <- w286 stop-if-true
          w287 = u32 1  # Yield Control
          n39 = shared-variable "My Computer\\Experiment_network_vars.lvlib\\Wait Loops"(w261, error in=w259) -> (error out=w258:errorcluster)
          n40 = Wait (ms)(milliseconds to wait=w287) -> ()  [unwired: 1 out]
          n41 = call-dynamic "get_data.vi"("error in (no error)"=w258, "Counter in"=w269) -> ("error out"=w266:errorcluster, 2:w257, "Counter out"=w268:refnum<class "Counter.lvclass">)  [unwired: 7 in]
          n42 = call-dynamic "plot1.vi"("error in (no error)"=w266, "Counter in"=w268) -> ("error out"=w265:errorcluster, "Counter out"=w267:refnum<class "Counter.lvclass">)  [unwired: 8 in]
          n43 = call-dynamic "is_done.vi"("error in (no error)"=w265, "HSDIO in"=w285) -> ("error out"=w281:errorcluster, "HSDIO is done?"=w273:bool, "HSDIO out"=w284:refnum<class "HSDIO.lvclass">)  [unwired: 7 in]
          n44 = call-dynamic "is_done.vi"("error in (no error)"=w281, "DAQmx_pulse_out in"=w283) -> ("error out"=w277:errorcluster, "task done?"=w272:bool, "DAQmx_pulse_out out"=w282:refnum<class "DAQmx_pulse_out.lvclass">)  [unwired: 7 in]
          n45 = call-dynamic "is_done.vi"("error in (no error)"=w277, "Analog_Output in"=w275) -> ("error out"=w276:errorcluster, "task done?"=w270:bool, "Analog_Output out"=w274:refnum<class "Analog_Output.lvclass">)  [unwired: 7 in]
          n46 = call-dynamic "check_timeout.vi"("error in (no error)"=w276, "ExperimentVariables in"=w260) -> ("error out"=w263:errorcluster, "timeout elapsed?"=w278:bool, "ExperimentVariables out"=w280:refnum<class "ExperimentVariables.lvclass">)  [unwired: 7 in]
          n47 = Compound Arithmetic op=AND(w273, w272, w270) -> (w271:bool)
          n48 = shared-variable "My Computer\\Experiment_network_vars.lvlib\\Stop"(error in=w263) -> (w264:bool, error out=w262:errorcluster)
          n49 = Unbundle By Name(w262) -> ("status"=w279:bool)
          n50 = Compound Arithmetic op=OR(w271, w264, w278, w279) -> (w286:bool)
        }
        n51 = call-dynamic "TTL_check.vi"("error in (no error)"=w208, "TTL_input in"=w202) -> ("error out"=w207:errorcluster, 1:w201, "TTL_input out"=w209:refnum<class "TTL_input.lvclass">)  [unwired: 7 in]
        n52 = Not Or "lasers were okay?"(1:w200, 2:w201) -> (0:w199:bool)
        n53 = call-dynamic "plot2.vi"("error in (no error)"=w207, "Counter in"=w229) -> ("error out"=w227:errorcluster, "Counter out"=w228:refnum<class "Counter.lvclass">)  [unwired: 8 in]
        n54 = call "stop_tasks.vi"("Counter (in)"=w228, "Analog_Output (in)"=w238, "HSDIO (in)"=w252, "DAQmx_pulse_out (in)"=w244, "error in"=w227) -> ("Counter"=w247:refnum<class "Counter.lvclass">, "Analog_Output"=w237:refnum<class "Analog_Output.lvclass">, "HSDIO"=w251:refnum<class "HSDIO.lvclass">, "DAQmx_pulse"=w243:refnum<class "DAQmx_pulse_out.lvclass">, "error out"=w233:errorcluster)  [unwired: 10 in]
        n55 = call-dynamic "acquire.vi"("Current Measurement"=w196, "Current Iteration"=w197, "error in (no error)"=w233, "ExperimentVariables (in)"=w232, "Hamamatsu_C9100-13 in"=w234) -> ("error out"=w231:errorcluster, "Array of ROI sums"=w213:dbl[][], "ExperimentVariables"=w222:refnum<class "ExperimentVariables.lvclass">, "Hamamatsu_C9100-13 out"=w223:refnum<class "Hamamatsu_C9100-13.lvclass">, "Image Array"=w225:T39[])  [unwired: 2 in]
        n56 = property on="Set Recent Image Array" class="Arr (strict)"(reference=w219, error in=w231, "Value"=w225) -> (error out=w216:errorcluster)  [unwired: 1 out]
        n57 = call "measurement_chart.vi"("error in"=w216, "Array of ROI"=w213, "Measurement Chart Settings"=w214, "Measurement Chart"=w217) -> ("error out"=w215:errorcluster)  [unwired: 7 in]
        n58 = call-dynamic "Read Run Test Mode.vi"("error in (no error)"=w215, "ExperimentVariables in"=w222) -> ("error out"=w220:errorcluster, "Run Test Mode"=w226:bool, "ExperimentVariables out"=w221:refnum<class "ExperimentVariables.lvclass">)  [unwired: 7 in]
        "Run Test Mode" <- w226
        n59 = call "filters.vi"("Counter Data"=w206, "error in"=w220, "lasers okay?"=w199, "Array of ROI sums"=w213, "Filter Cluster"=w218) -> ("error out"=w230:errorcluster, "All shots passed filters?"=w198:bool)  [unwired: 5 in]
        n60 = call "pause_after_measurement.vi"("error in (no error)"=w230) -> ("error out"=w211:errorcluster)  [unwired: 10 in]
        n61 = shared-variable "My Computer\\Experiment_network_vars.lvlib\\Stop"(error in=w211) -> (w212:bool, error out=w210:errorcluster)
        n62 = case "If in Run Test Mode,\ndon't create large image array." shown="False" w226 {
          tunnel: w225 -> [w256 _]
          tunnel: [w256 _] -> w224
          frame False {
          }
          frame True {
          }
        }
        n63 = Unbundle By Name(w210) -> ("status"=w255:bool)
        n64 = Compound Arithmetic op=OR(w198, w212, w255) -> (w254:bool)
      }
      n65 = call "save_data.vi"("Array of ROI sums"=w185, "Current Measurement"=w163, "error in (no error)"=w182, "ExperimentVariables (in)"=w183, "Counter (in)"=w181, "Camera (in)"=w179) -> ("error out"=w172:errorcluster, "ExperimentVariables"=w177:refnum<class "ExperimentVariables.lvclass">, "Counter"=w180:refnum<class "Counter.lvclass">, "Camera"=w178:refnum<class "Hamamatsu_C9100-13.lvclass">)  [unwired: 2 in]
      n66 = shared-variable "My Computer\\Experiment_network_vars.lvlib\\Stop"(error in=w172) -> (w171:bool, error out=w170:errorcluster)
      n67 = Unbundle By Name(w170) -> ("status"=w192:bool)
      n68 = Or(x=w192, y=w171) -> (x .or. y?=w191:bool)
    }
    n69 = call-dynamic "close_iteration_data_files.vi"("error in (no error)"=w127, "Hamamatsu_C9100-13 (in)"=w123, "Counter (in)"=w122, "ExperimentVariables in"=w125) -> ("error out"=w126:errorcluster, "Hamamatsu_C9100-13"=w112:refnum<class "Hamamatsu_C9100-13.lvclass">, "Counter out"=w121:refnum<class "Counter.lvclass">, "ExperimentVariables out"=w124:refnum<class "ExperimentVariables.lvclass">)  [unwired: 4 in]
    n70 = call-dynamic "close.vi"("error in (no error)"=w126, "DAQmx_pulse_out in"=w149) -> ("error out"=w148:errorcluster)  [unwired: 8 in, 1 out]
    n71 = call-dynamic "remove_waveforms.vi"("error in (no error)"=w148, "HSDIO in"=w156) -> ("error out"=w139:errorcluster, "HSDIO out"=w155:refnum<class "HSDIO.lvclass">)  [unwired: 8 in]
    n72 = call-dynamic "close.vi"("error in (no error)"=w139, "Analog_Output in"=w140) -> ("error out"=w110:errorcluster)  [unwired: 8 in, 1 out]
    n73 = call "iteration_graph_update.vi"("Iteration Graph Settings"=w108, "error in (no error)"=w110, "Iteration Number"=w85, "ROI Array In"=w111, "GUI refnum cluster"=w101) -> ("error out"=w109:errorcluster)  [unwired: 5 in, 1 out]
    n74 = call "pause_after_iteration.vi"("error in (no error)"=w109) -> ("error out"=w90:errorcluster)  [unwired: 10 in]
    n75 = shared-variable "My Computer\\Experiment_network_vars.lvlib\\Stop"(error in=w90) -> (w91:bool, error out=w89:errorcluster)
    n76 = Unbundle By Name(w90) -> ("status"=w161:bool)
    n77 = Or(x=w161, y=w91) -> (x .or. y?=w162:bool)
  }
  "Image Array for whole experiment" <- w74
  "Array of ROI sums" <- w67
  n78 = call-dynamic "get_Photoelectron_scaling.vi"("error in (no error)"=w33, "Hamamatsu_C9100-13 in"=w34) -> ("error out"=w32:errorcluster, "Photoelectron Scaling"=w30:dbl, "Hamamatsu_C9100-13 out"=w31:refnum<class "Hamamatsu_C9100-13.lvclass">)  [unwired: 7 in]
  n79 = call-dynamic "Read timestamped data path.vi"("error in (no error)"=w32, "ExperimentVariables in"=w50) -> ("error out"=w48:errorcluster, "Specific Data Files Path"=w10:path, "ExperimentVariables out"=w37:refnum<class "ExperimentVariables.lvclass">)  [unwired: 7 in]
  n80 = call "make_histogram.vi"("# intervals (mutli-shot)"="# intervals (mutli-shot)", "Array of ROI sums"=w67, "Photoelectron Scaling"=w30) -> ("Histogram over all images, for each region"=→"Histogram of ROI Sum over All Images for last ROI":T42)
  n81 = call "save_comments.vi"("error in"=w48, "Str Refnum"="Notes Refnum", "base path"=w10) -> ("error out"=w38:errorcluster)  [unwired: 8 in]
  n82 = call "average_images.vi"("error in (no error)"=w38, "Hamamatsu_C9100-13 (in)"=w31) -> ("error out"=w40:errorcluster, "Hamamatsu_C9100-13 out"=w68:refnum<class "Hamamatsu_C9100-13.lvclass">, "Average of Images"=w42:T39)  [unwired: 7 in]
  n83 = call-dynamic "Read Run Test Mode.vi"("error in (no error)"=w40, "ExperimentVariables in"=w37) -> ("error out"=w43:errorcluster, "Run Test Mode"=w44:bool, "ExperimentVariables out"=w39:refnum<class "ExperimentVariables.lvclass">)  [unwired: 7 in]
  n84 = case shown="False" w44 {
    tunnel: w43 -> [w289 w297]
    tunnel: w42 -> [w293 w298]
    tunnel: [w292 w298] -> w41
    tunnel: [w294 w297] -> w13
    tunnel: w39 -> [w291 w296]
    tunnel: [w295 w296] -> w36
    frame False {
      n85 = call "save_avg_image.vi"("error in (no error)"=w289, "Image"=w293, "ExperimentVariables in"=w291) -> ("error out"=w288:errorcluster, "Image Out (duplicate)"=w292:T39, "ExperimentVariables out"=w290:refnum<class "ExperimentVariables.lvclass">)  [unwired: 6 in]
      n86 = call "save_log.vi"("error in"=w288, "ExperimentVariables in"=w290) -> ("error out"=w294:errorcluster, "ExperimentVariables out"=w295:refnum<class "ExperimentVariables.lvclass">)  [unwired: 8 in]
    }
    frame True {
    }
  }
  "Average of All Images from experiment" <- w41
  n87 = call "move_andor_files.vi"("error in"=w13, "Data Files Path"=w10, "Andor setup"=w11) -> ("error out"=w12:errorcluster)  [unwired: 8 in]
  n88 = call-dynamic "upload_data.vi"("error in (no error)"=w12, "ExperimentVariables in"=w36) -> ("error out"=w35:errorcluster)  [unwired: 8 in, 1 out]
  n89 = call "close_tasks.vi"("Counter (in)"=w77, "HSDIO (in)"=w76, "Camera (in)"=w68, "TTL_input in"=w1, "error in"=w35) -> ("Counter"=→"Counter out":refnum<class "Counter.lvclass">, "HSDIO"=→"HSDIO":refnum<class "HSDIO.lvclass">, "Camera"=→"Camera out":refnum<class "Hamamatsu_C9100-13.lvclass">, "error out"=w78:errorcluster)  [unwired: 10 in, 1 out]
  n90 = call "setup_gui.vi"("Enum"=T40."experiment end", "GUI refnum cluster"="GUI refnum cluster", "error in (no error)"=w78) -> ("error out"=w56:errorcluster)  [unwired: 12 in]
  n91 = call "append_to_log.vi"("error in"=w56, "string"="Experiment ended") -> ("error out"=→"error out":errorcluster)  [unwired: 9 in]
